vi "DAQ.Start.vi"(8 "error in (no error)":errorcluster, 11 "Instrument.DAQ in":refnum<class "Instrument.DAQ.lvclass">) -> (0 "error out":errorcluster, 3 "Instrument.DAQ out":refnum<class "Instrument.DAQ.lvclass">)   [LabVIEW 2019, in "Instrument.Lockin.lvlib" / "Instrument.DAQ.lvclass"]
uses:
  Instrument.DAQ.lvclass
  DAQmx/DAQmx.lvclass
  Typedefs/Sweep.State--enum.ctl
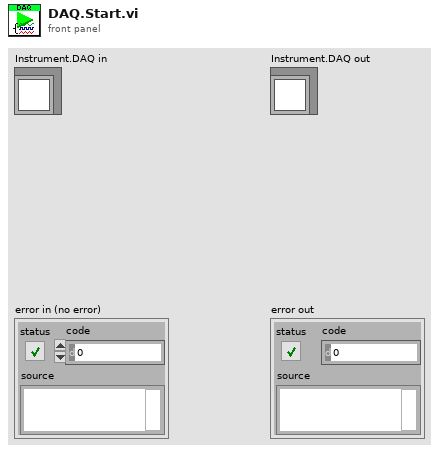
[diagram p1: front panel]
types:
  T1 = typedef "Instrument.Lockin.lvlib/Instrument.DAQ.lvclass/Sweep.State--enum.ctl" = enum16{"idle", "initialize", "wait", "sweep", "stop"}
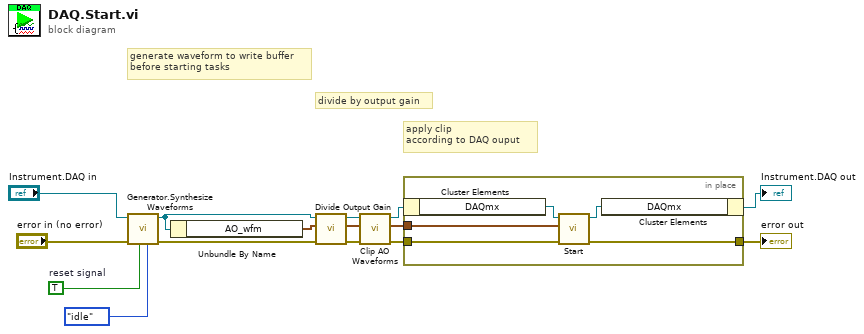
[diagram p0: block diagram]
diagram:
  w14 = TRUE  # reset signal
  # "apply clip\naccording to DAQ ouput"
  # "divide by output gain"
  # "generate waveform to write buffer\nbefore starting tasks"
  n1 = call "Generator.Synthesize Waveforms.vi"("sweep state"=Sweep.State--enum."idle", "Reset Phase?"=w14, "error in (no error)"="error in (no error)", "Instrument.DAQ"="Instrument.DAQ in") -> ("error out"=w8:errorcluster, "Instrument.DAQ"=w10:refnum<class "Instrument.DAQ.lvclass">)  [unwired: 6 in]
  n2 = Unbundle By Name(w10) -> ("AO_wfm"=w9:waveform(dbl)[])
  n3 = call "Divide Output Gain.vi"("error in (no error)"=w8, "WFM in"=w9, "Instrument.DAQ"=w10) -> ("error out"=w11:errorcluster, "WFM out"=w13:waveform(dbl)[], "Instrument.DAQ out"=w12:refnum<class "Instrument.DAQ.lvclass">)  [unwired: 6 in]
  n4 = call "Clip AO Waveforms.vi"("error in (no error)"=w11, "AO []"=w13, "Instrument.DAQ in"=w12) -> ("error out"=w7:errorcluster, "Clipped AO []"=w4:waveform(dbl)[], "Instrument.DAQ out"=w2:refnum<class "Instrument.DAQ.lvclass">)  [unwired: 6 in]
  n5 = in-place {
    in-place-border: w7 -> [w20]
    in-place-border: [w19] -> w5
    in-place-border: w4 -> [w18]
    n6 = in-place-cluster #1(w2) -> ("DAQmx"=w17:refnum<class "DAQmx.lvclass">)
    n7 = call "Start.vi"("error in"=w20, "WFM in"=w18, "DAQmx in"=w17) -> ("error out"=w19:errorcluster, "DAQmx out"=w16:refnum<class "DAQmx.lvclass">)  [unwired: 7 in]
    n8 = in-place-cluster #1("DAQmx"=w16) -> (→"Instrument.DAQ out":refnum<class "Instrument.DAQ.lvclass">)
  }
  "error out" <- w5
